vi "Update Child.vi"(8 "error in (no error)":errorcluster, 11 "Package in":refnum<class "Package.lvclass">) -> (0 "error out":errorcluster, 3 "Package out":refnum<class "Package.lvclass">)   [LabVIEW 2020, in "neg-pkg.lvlib" / "Package.lvclass"]
uses:
  Package.lvclass
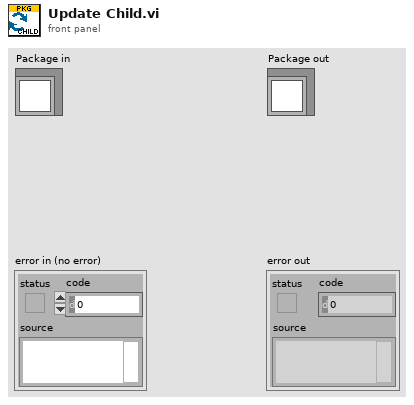
[diagram p1: front panel]
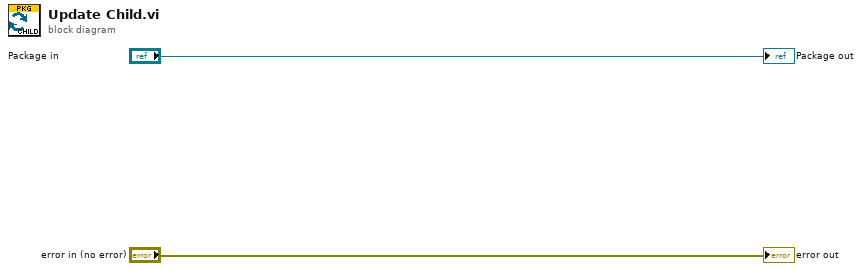
[diagram p0: block diagram]
diagram:
  "error out" <- "error in (no error)"
  "Package out" <- "Package in"
